vi "Proyecto Puntos extra Adrian Morales.vi"() -> ()   [LabVIEW 2025]
uses:
  <vilib>/MakerHub/LINX/Public/Peripherals/Digital/Digital Read 1 Chan.vi
  <vilib>/MakerHub/LINX/Public/Peripherals/Analog/Analog Read 1 Chan.vi
  <vilib>/MakerHub/LINX/Public/Peripherals/Digital/Digital Read N Chans.vi
  <vilib>/MakerHub/LINX/Public/Peripherals/Analog/Analog Read N Chans.vi
  <vilib>/MakerHub/LINX/Private/Local IO/LinxDigitalRead.vi
  <vilib>/MakerHub/LINX/Public/Utilities/Check Channel.vi
  <vilib>/MakerHub/LINX/Private/Local IO/LinxAnalogRead.vi
  <vilib>/MakerHub/LINX/Public/Utilities/Open Serial.vi
  <vilib>/MakerHub/LINX/Private/Utilties/Generate Error.vi
  <vilib>/MakerHub/LINX/LMH-LINX.lvlib
panel:
  out "CASETA":string
  in  "Serial Port":refnum<visa-resource-name>="N/A"
  out "TICKET":bool
  out "ESPERE":bool
  out "Siga":bool
  in  "stop":bool
  out "Barrera Abierta":bool
  out "Plaza Ocupada":bool
  out "Plaza Libre":bool
  out "Barrera Cerrada":bool
  # "SISTEMA DE CABINADE ESTACINAMIENTO"
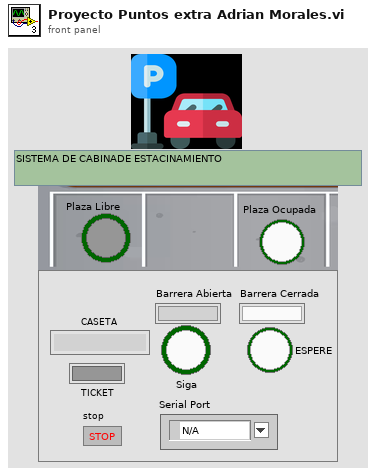
[diagram p1: front panel]
types:
  T1 = typedef "LMH-LINX.lvlib/LINX Ref.ctl" = cluster{"IO":T2, "Interface":T3, "LINX Device Config":T4}
  T2 = typedef "LMH-LINX.lvlib/Platform.ctl" = enum16{"Remote", "Local"}
  T3 = typedef "LMH-LINX.lvlib/Interface.ctl" = enum16{"Serial", "TCP"}
  T4 = typedef "LMH-LINX.lvlib/Device.lvlib/LINX Device Config.ctl" = cluster{"Interface":T3, "COM Port":refnum<visa-resource-name>, "TCP Configuration":T5, "Device Family":u8, "Device ID":u8, "Device Name":string, "TCP Ref":refnum<k5>, "Channels":T6}
  T5 = typedef "LMH-LINX.lvlib/Device.lvlib/TCP Config.ctl" = cluster{"IP Address":string, "Port":u16}
  T6 = typedef "LMH-LINX.lvlib/Channels.ctl" = cluster{"DI":u8[], "DO":u8[], "AI":u8[], "AO":u8[], "PWM":u8[], "QE":u8[], "UART":u8[], "I2C 2":u8[], "SPI":u8[], "CAN":u8[], "Servo":u8[], "AI Ref (V)":dbl, "AI Resolution (Bits)":u8, "AO Ref (V)":dbl, "AO Resolution (Bits)":u8}
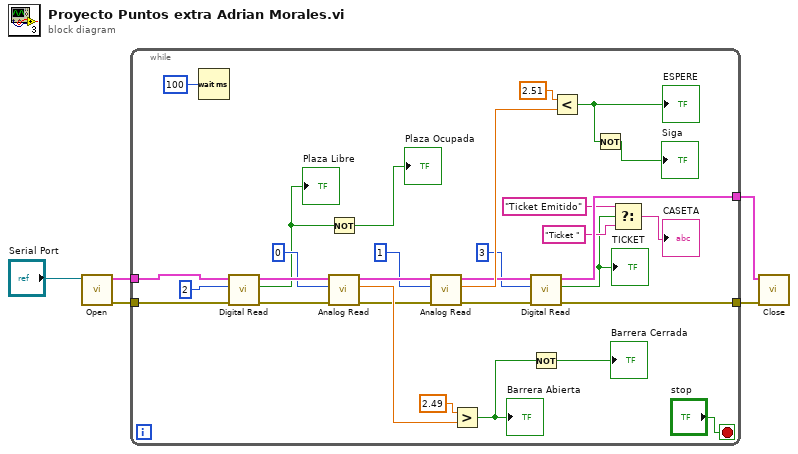
[diagram p0: block diagram]
diagram:
  n1 = call-poly <vilib>:"Open.vi"("Serial Port"="Serial Port") -> ("Error Out"=w4:errorcluster, "LINX Resource"=w5:T1)  [unwired: 8 in, 1 out]
  n2 = while {
    tunnel: w5 -> [w33]
    tunnel: w4 -> [w32]
    tunnel: [w17] -> w3
    tunnel: [w15] -> w2
    stop <- "stop" stop-if-true
    n3 = Wait (ms)(milliseconds to wait=u32 100) -> ()  [unwired: 1 out]
    n4 = call-poly <vilib>:"Digital Read.vi"("Error In"=w32, "DI Channel"=u8 2, "LINX Resource"=w33) -> ("Error Out"=w31:errorcluster, "DI Value"=w23:bool, "LINX Resource"=w30:T1)  [unwired: 6 in]
    "Plaza Libre" <- w23
    n5 = Not(x=w23) -> (.not. x?=→"Plaza Ocupada":bool)
    n6 = call-poly <vilib>:"Analog Read.vi"("Error In"=w31, "Analog Channel"=u8 0, "LINX Resource"=w30) -> ("Error Out"=w21:errorcluster, "Voltage"=w27:dbl, "LINX Resource"=w22:T1)  [unwired: 5 in, 1 out]
    n7 = call-poly <vilib>:"Analog Read.vi"("Error In"=w21, "Analog Channel"=u8 1, "LINX Resource"=w22) -> ("Error Out"=w14:errorcluster, "Voltage"=w19:dbl, "LINX Resource"=w16:T1)  [unwired: 5 in, 1 out]
    n8 = Greater?(x=2.49, y=w27) -> (0:w25:bool)
    "Barrera Abierta" <- w25
    n9 = call-poly <vilib>:"Digital Read.vi"("Error In"=w14, "DI Channel"=u8 3, "LINX Resource"=w16) -> ("Error Out"=w15:errorcluster, "DI Value"=w9:bool, "LINX Resource"=w17:T1)  [unwired: 6 in]
    "TICKET" <- w9
    n10 = Not(x=w25) -> (.not. x?=→"Barrera Cerrada":bool)
    n11 = Less?(x=2.51, y=w19) -> (x < y?=w6:bool)
    "ESPERE" <- w6
    n12 = Not(x=w6) -> (.not. x?=→"Siga":bool)
    n13 = Select(t="Ticket Emitido", s=w9, f="Ticket ") -> (s? t:f=→"CASETA":string)
  }
  n14 = call <vilib>:"Close.vi"("Error In"=w2, "LINX Resource"=w3) -> ()  [unwired: 9 in, 1 out]
